vi "is_developer.vi"(8 "error in (no error)":errorcluster) -> (0 "error out":errorcluster, 1 "svn version number":string, 2 "is developer?":bool)   [LabVIEW 2010, in "HelioUpdateMH100803.lvclass"]
uses:
  HelioUpdateMH100803.lvclass
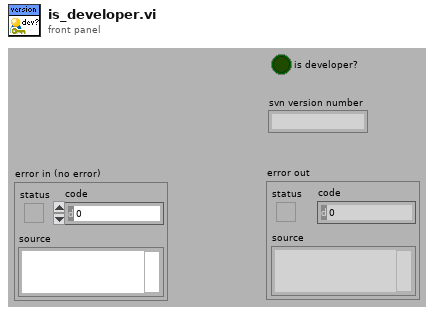
[diagram p1: front panel]
types:
  T1 = enum16{"open", "replace", "create", "open or create", "replace or create", "replace or create with confirmation"}
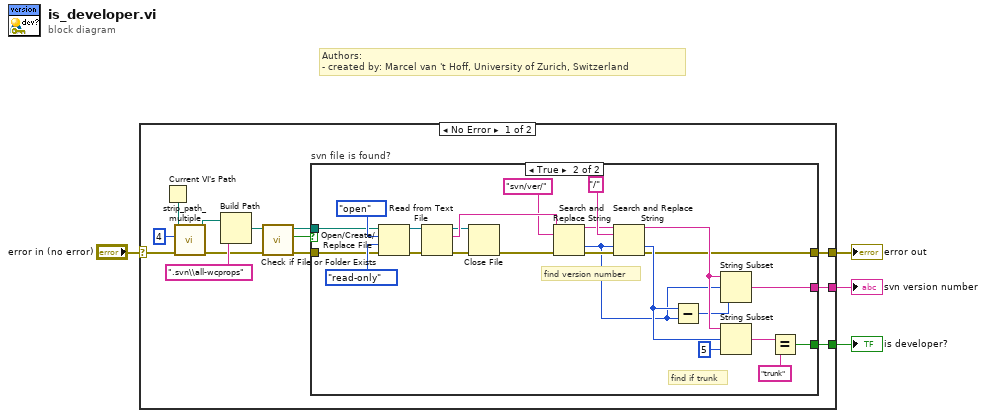
[diagram p0: block diagram]
diagram:
  # "Authors: \n- created by: Marcel van 't Hoff, University of Zurich, Switzerland"
  n1 = case shown="No Error" "error in (no error)" {
    selector: "error in (no error)" -> [w12 w43]
    tunnel: [w17 _] -> w4
    tunnel: [w15 _] -> w3
    tunnel: [w13 w43] -> w2
    frame No Error {
      n2 = Current VI's Path() -> (path=w14:path)
      n3 = call "strip_path_multiple.vi"("error in (no error)"=w12, "number of strips"=4, "path in"=w14) -> ("error out"=w6:errorcluster, "path out"=w7:path)  [unwired: 7 in]
      n4 = Build Path(base path=w7, name or relative path=".svn\\all-wcprops") -> (appended path=w5:path)
      n5 = call <vilib>:"Check if File or Folder Exists.vi"("error in (no error)"=w6, "path"=w5) -> ("error out"=w10:errorcluster, "file or folder exists?"=w9:bool, "dup path"=w11:path)  [unwired: 7 in]
      n6 = case "svn file is found?" shown="True" w9 {
        tunnel: [_ w42] -> w17
        tunnel: [_ w33] -> w15
        tunnel: [w18 w21] -> w13
        tunnel: w11 -> [_ w19]
        tunnel: w10 -> [w18 w20]
        frame False {
        }
        frame True {
          # "find if trunk"
          # "find version number"
          n7 = Open/Create/Replace File(file path (use dialog)=w19, error in=w20, operation (0:open)=T1."open", access (0:read/write)=enum16{"read/write", "read-only", "write-only"}."read-only") -> (refnum out=w24:refnum<file>, error out=w25:errorcluster)  [unwired: 2 in, 1 out]
          n8 = Read from Text File(file (use dialog)=w24, error in=w25) -> (refnum out=w26:refnum<file>, text=w34:string, error out=w27:errorcluster)  [unwired: 2 in, 1 out]
          n9 = Close File(refnum=w26, error in=w27) -> (error out=w38:errorcluster)  [unwired: 1 out]
          n10 = Search and Replace String(input string=w34, search string="svn/ver/", error in=w38) -> (result string=w29:string, offset past replacement=w31:i32, error out=w39:errorcluster)  [unwired: 5 in, 1 out]
          n11 = Search and Replace String(input string=w29, search string="/", offset=w31, error in=w39) -> (result string=w35:string, offset past replacement=w37:i32, error out=w21:errorcluster)  [unwired: 4 in, 1 out]
          n12 = Subtract(x=w37, y=w31) -> (x-y=w32:i32)
          n13 = String Subset(string=w35, offset (0)=w31, length (rest)=w32) -> (substring=w33:string)
          n14 = String Subset(string=w35, offset (0)=w37, length (rest)=5 ("length (rest)")) -> (substring=w40:string)
          n15 = Equal?(x=w40, y="trunk") -> (x = y?=w42:bool)
        }
      }
    }
    frame Error {
    }
  }
  "error out" <- w2
  "svn version number" <- w3
  "is developer?" <- w4
